vi "Get Phasor Scaling.vi"(11 "Phasor Configuration":T2) -> (3 "Phasor Scaling":T1)   [LabVIEW 2013, in "PMU Recorder Light.lvlib" / "Statnett C37.118 DLL.lvclass"]
uses:
  Statnett C37.118 DLL.lvclass
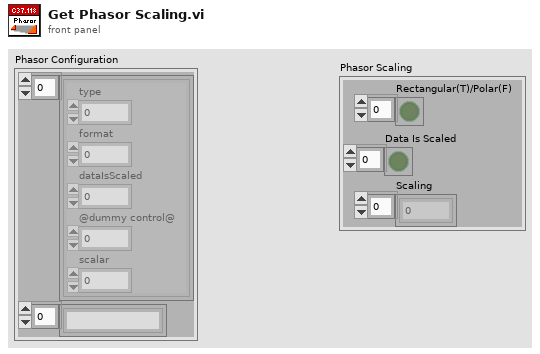
[diagram p1: front panel]
types:
  T1 = cluster{"Rectangular(T)/Polar(F)":bool[], "Data Is Scaled":bool[], "Scaling":sgl[]}
  T2 = cluster{cluster{"type":u8, "format":u8, "dataIsScaled":u8, "@dummy control@":i8, "scalar":sgl}[], string[]}
  T3 = cluster{"type":u8, "format":u8, "dataIsScaled":u8, "@dummy control@":i8, "scalar":sgl}[]
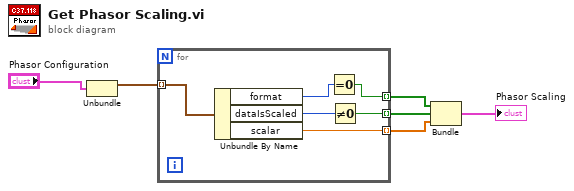
[diagram p0: block diagram]
diagram:
  n1 = Unbundle("Phasor Configuration") -> (w5:T3)  [unwired: 1 out]
  n2 = for {
    tunnel: w5 -> [w12] mode=indexing
    tunnel: [w10] -> w3 mode=indexing
    tunnel: [w7] -> w4 mode=indexing
    tunnel: [w9] -> w2 mode=indexing
    n3 = Unbundle By Name(w12) -> ("format"=w8:u8, "dataIsScaled"=w11:u8, "scalar"=w9:sgl)
    n4 = Equal To 0?(x=w8) -> (x = 0?=w7:bool)
    n5 = Not Equal To 0?(x=w11) -> (x != 0?=w10:bool)
  }
  n6 = Bundle(w4, w3, w2) -> (→"Phasor Scaling":cluster{bool[], bool[], sgl[]})  [unwired: 1 in]
